vi "test Add-Find-Remove Messages.vi"(8 "error in":errorcluster, 11 "TestCase in":refnum<class "Scripting.lvclass">) -> (0 "error out":errorcluster, 3 "TestCase out":refnum<class "Scripting.lvclass">)   [LabVIEW 2020, in "Scripting.lvclass"]
uses:
  Scripting.lvclass
  C:/Git/niveristand-custom-device-testing-tools/VeriStandScriptingTestCase/VeriStandScriptingTestCase.lvclass
  Shared/1553 Channel.ctl
  Shared/Terminal Name and Address.ctl
  Shared/Address.ctl
  Shared/Message Definition.ctl
  Shared/Message Type.ctl
  Shared/Terminal Endpoint.ctl
  Shared/Parameter Definition.ctl
  niveristand-custom-device-testing-tools/VeriStandScriptingTestCase/VeriStandScriptingTestCase.lvclass/VeriStandScriptingTestCase.ctl
  niveristand-custom-device-testing-tools/VeriStandScriptingTestCase/Read Target.vi
  NationalInstruments.VeriStand.SystemDefinitionAPI
  <vilib>/addons/_JKI Toolkits/VI Tester/TestCase.llb/TestCase.lvclass
  Scripting/Ballard MIL-STD-1553 Scripting.lvlib
  C:/Program Files (x86)/National Instruments/LabVIEW 2020/vi.lib/addons/_JKI Toolkits/VI Tester/TestCase.llb/TestCase.lvclass
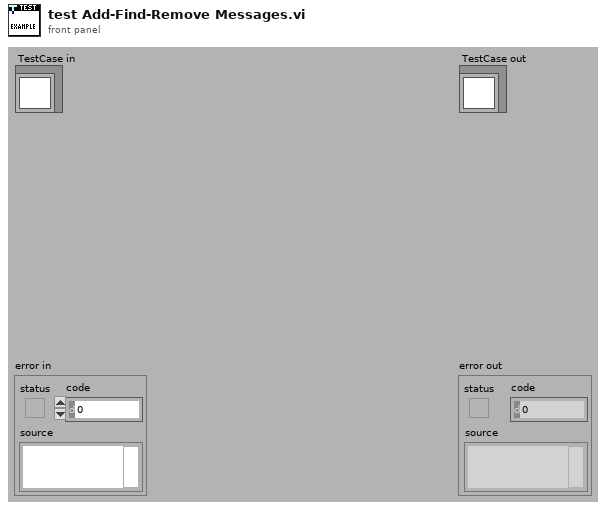
[diagram p1: front panel]
types:
  T1 = typedef "1553 Channel.ctl" = cluster{"HW channel":u16, "terminals":T2[], "messages":T4[], "acyclic frame names":string[]}
  T2 = typedef "Terminal Name and Address.ctl" = cluster{"name":string, "terminal address":T3}
  T3 = typedef "Address.ctl" = u16
  T4 = typedef "Message Definition.ctl" = cluster{"name":string, "message type":T5, "endpoint Rx":T6, "endpoint Tx":T6, "mode code":u16, "number of words":u16, "parameters":cluster{"name":string, "default value":dbl, "unit":string, "parameter definition":T7}[], "create timestamp channel":bool}
  T5 = typedef "Message Type.ctl" = string
  T6 = typedef "Terminal Endpoint.ctl" = cluster{"terminal address":T3, "subaddress":T3}
  T7 = typedef "Parameter Definition.ctl" = cluster{"start index":i32, "size (bits)":i32, "encoding":enum16{"BNR", "BCD", "Discrete"}, "signed":bool, "multiplier":dbl, "offset":dbl}
  T8 = typedef "Custom Device API.lvlib/Custom Device Item Ref.ctl" = u64
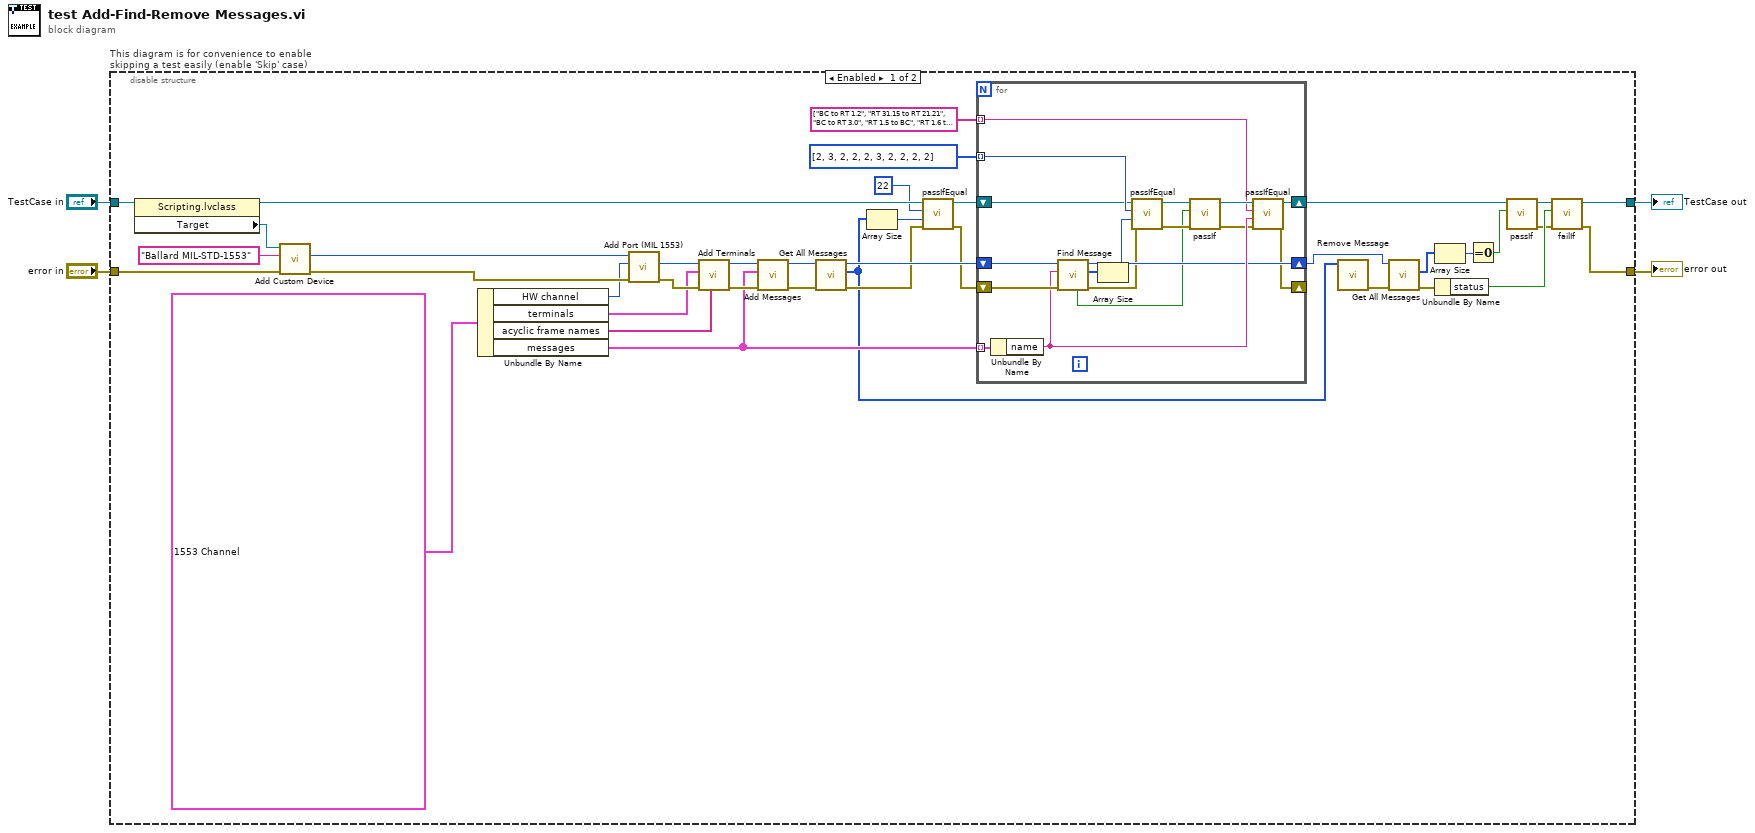
[diagram p0: block diagram]
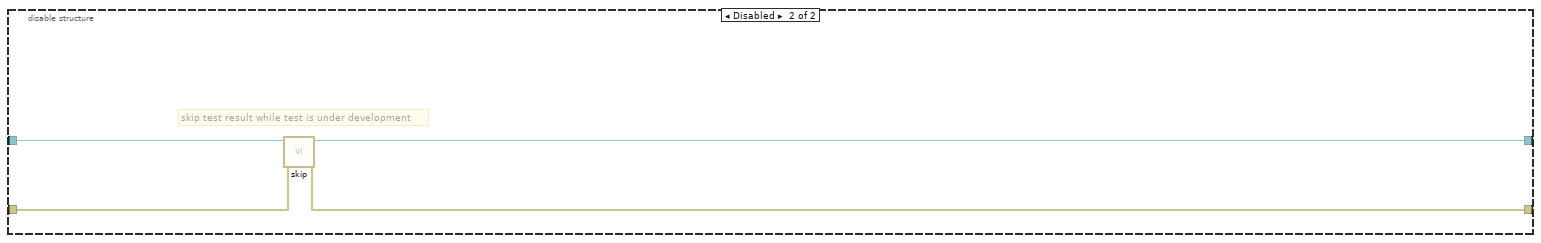
[diagram p2: hidden frame]
diagram:
  n1 = disable-structure "This diagram is for convenience to enable skipping a test easily (enable 'Skip' case)" shown="Enabled" {
    disable-tunnel: "TestCase in" -> [w41 w65]
    disable-tunnel: [w38 w63] -> w1
    disable-tunnel: [w39 w64] -> w3
    disable-tunnel: "error in" -> [w43 w62]
    frame Enabled {
      n2 = property class="Scripting.lvclass"(reference=w41) -> (reference out=w24:refnum<class "Scripting.lvclass">, "Target"=w40:refnum<k24>)  [unwired: 1 in, 1 out]
      n3 = call "Add Custom Device.vi"("error in"=w43, "name"="Ballard MIL-STD-1553", "target in"=w40) -> ("error out"=w36:errorcluster, "Ballard MIL-STD-1553 custom device"=w35:T8)  [unwired: 6 in, 1 out]
      n4 = Unbundle By Name(T1 {"HW channel"=0, "terminals"=[{"name"="Bus Controller", "terminal address"=0}, {"name"="Remote Terminal 1", "terminal address"=1}, {"name"="Remote Terminal 15", "terminal address"=15}, {"name"="Remote Terminal 21", "terminal address"=21}, {"name"="Remote Terminal 31 (Broadcast)", "terminal address"=31}], "messages"=[{"name"="BC to RT 1.2", "message type"="BC to RT", "endpoint Rx"={"terminal address"=1, "subaddress"=2}, "endpoint Tx"={"terminal address"=0, "subaddress"=0}, "mode code"=0, "number of words"=3, "parameters"=[], "create timestamp channel"=FALSE}, {"name"="RT 31.15 to RT 21.21", "message type"="RT to RT", "endpoint Rx"={"terminal address"=31, "subaddress"=21}, "endpoint Tx"={"terminal address"=15, "subaddress"=21}, "mode code"=0, "number of words"=11, "parameters"=[], "create timestamp channel"=FALSE}, {"name"="BC to RT 3.0", "message type"="BC to RT", "endpoint Rx"={"terminal address"=1, "subaddress"=3}, "endpoint Tx"={"terminal address"=0, "subaddress"=0}, "mode code"=0, "number of words"=4, "parameters"=[], "create timestamp channel"=FALSE}, {"name"="RT 1.5 to BC", "message type"="RT to BC", "endpoint Rx"={"terminal address"=0, "subaddress"=0}, "endpoint Tx"={"terminal address"=1, "subaddress"=5}, "mode code"=0, "number of words"=6, "parameters"=[], "create timestamp channel"=FALSE}, {"name"="RT 1.6 to BC", "message type"="RT to BC", "endpoint Rx"={"terminal address"=0, "subaddress"=0}, "endpoint Tx"={"terminal address"=1, "subaddress"=6}, "mode code"=0, "number of words"=2, "parameters"=[], "create timestamp channel"=FALSE}, {"name"="RT 15.20 to RT 1.20", "message type"="RT to RT", "endpoint Rx"={"terminal address"=15, "subaddress"=20}, "endpoint Tx"={"terminal address"=1, "subaddress"=20}, "mode code"=0, "number of words"=4, "parameters"=[], "create timestamp channel"=FALSE}, {"name"="MC 16", "message type"="MC", "endpoint Rx"={"terminal address"=0, "subaddress"=0}, "endpoint Tx"={"terminal address"=1, "subaddress"=31}, "mode code"=16, "number of words"=1, "parameters"=[], "create timestamp channel"=FALSE}, {"name"="MC 17", "message type"="MC", "endpoint Rx"={"terminal address"=1, "subaddress"=31}, "endpoint Tx"={"terminal address"=0, "subaddress"=0}, "mode code"=17, "number of words"=1, "parameters"=[], "create timestamp channel"=FALSE}, {"name"="BC to RT 31.28", "message type"="BC to RT", "endpoint Rx"={"terminal address"=31, "subaddress"=28}, "endpoint Tx"={"terminal address"=0, "subaddress"=0}, "mode code"=0, "number of words"=6, "parameters"=[], "create timestamp channel"=FALSE}, {"name"="MC 1", "message type"="MC", "endpoint Rx"={"terminal address"=31, "subaddress"=31}, "endpoint Tx"={"terminal address"=0, "subaddress"=0}, "mode code"=1, "number of words"=0, "parameters"=[], "create timestamp channel"=FALSE}], "acyclic frame names"=["acyclicFrame ID56"]} ("1553 channel")) -> ("HW channel"=w33:u16, "terminals"=w28:T2[], "acyclic frame names"=w27:string[], "messages"=w21:T4[])
      n5 = call "Add Port (MIL 1553).vi"("error in"=w36, "port number"=w33, "Ballard MIL-STD 1553 custom device in"=w35) -> ("error out"=w31:errorcluster, "port"=w32:T8)  [unwired: 6 in, 1 out]
      n6 = call "Add Terminals.vi"("acyclic frame names"=w27, "error in"=w31, "terminals"=w28, "port in"=w32) -> ("error out"=w29:errorcluster, "port out"=w30:T8)  [unwired: 6 in]
      n7 = call "Add Messages.vi"("error in"=w29, "messages"=w21, "port in"=w30) -> ("error out"=w25:errorcluster, "port out"=w34:T8)  [unwired: 7 in]
      n8 = call "Get All Messages.vi"("error in"=w25, "port in"=w34) -> ("error out"=w19:errorcluster, "messages"=w17:T8[], "port out"=w22:T8)  [unwired: 7 in]
      n9 = Array Size(array=w17) -> (size(s)=w23:i32)
      n10 = call-dynamic "passIfEqual.vi"("error in (no error)"=w19, "y"=w23, "x"=22 ("size(s)"), "TestCase in"=w24) -> ("error out"=w18:errorcluster, "TestCase out"=w5:refnum<class "Scripting.lvclass">)  [unwired: 6 in]
      n11 = for {
        shift-right: [w45] -> _
        shift-left: w18 -> [w60]
        tunnel: w21 -> [w59] mode=indexing
        shift-right: [w56] -> w14
        shift-left: w22 -> [w61]
        tunnel: string[] ["BC to RT 1.2", "RT 31.15 to RT 21.21", "BC to RT 3.0", "RT 1.5 to BC", "RT 1.6 to BC", "RT 15.20 to RT 1.20", "MC 16", "MC 17", "BC to RT 31.28", "MC 1"] ("Array") -> [w51] mode=indexing
        tunnel: i32[] [2, 3, 2, 2, 2, 3, 2, 2, 2, 2] ("Array 3") -> [w50] mode=indexing
        shift-right: [w49] -> w6
        shift-left: w5 -> [w47]
        n12 = Unbundle By Name(w59) -> ("name"=w58:string)
        n13 = call "Find Message.vi"("error in"=w60, "message name"=w58, "port in"=w61) -> ("error out"=w46:errorcluster, "message refs"=w57:T8[], "port out"=w56:T8, "found?"=w44:bool)  [unwired: 5 in]
        n14 = Array Size(array=w57) -> (size(s)=w48:i32)
        n15 = call-dynamic "passIfEqual.vi"("error in (no error)"=w46, "y"=w48, "x"=w50, "TestCase in"=w47) -> ("error out"=w53:errorcluster, "TestCase out"=w52:refnum<class "Scripting.lvclass">)  [unwired: 6 in]
        n16 = call-dynamic "passIf.vi"("error in (no error)"=w53, "pass"=w44, "TestCase in"=w52) -> ("error out"=w55:errorcluster, "TestCase out"=w54:refnum<class "Scripting.lvclass">)  [unwired: 7 in]
        n17 = call-dynamic "passIfEqual.vi"("error in (no error)"=w55, "y"=w58, "x"=w51, "TestCase in"=w54) -> ("error out"=w45:errorcluster, "TestCase out"=w49:refnum<class "Scripting.lvclass">)  [unwired: 6 in]
      }
      n18 = call "Remove Message.vi"("message refs"=w17) -> ("error out"=w16:errorcluster)  [unwired: 10 in]
      n19 = call "Get All Messages.vi"("error in"=w16, "port in"=w14) -> ("error out"=w15:errorcluster, "messages"=w13:T8[])  [unwired: 7 in, 1 out]
      n20 = Array Size(array=w13) -> (size(s)=w12:i32)
      n21 = Unbundle By Name(w15) -> ("status"=w37:bool)
      n22 = Equal To 0?(x=w12) -> (x = 0?=w11:bool)
      n23 = call-dynamic "passIf.vi"("pass"=w11, "TestCase in"=w6) -> ("error out"=w9:errorcluster, "TestCase out"=w10:refnum<class "Scripting.lvclass">)  [unwired: 8 in]
      n24 = call-dynamic "failIf.vi"("error in (no error)"=w9, "fail"=w37, "TestCase in"=w10) -> ("error out"=w39:errorcluster, "TestCase out"=w38:refnum<class "Scripting.lvclass">)  [unwired: 7 in]
    }
    frame Disabled {
      # "skip test result while test is under development"
      n25 = call <vilib>:"skip.vi"("error in (no error)"=w62, "TestCase in"=w65) -> ("error out"=w64:errorcluster, "TestCase out"=w63:refnum<class "Scripting.lvclass">)  [unwired: 8 in]
    }
  }
  "error out" <- w3
  "TestCase out" <- w1
